vi "MotionMagicVoltage SetControl.vi"(0 "LimitReverseMotion":bool, 1 "FeedForward":dbl, 2 "OverrideBrakeDurNeutral":bool, 3 "Update Frequency (Hz)":dbl=100.0, 5 "StopSendingOtherRequests":bool=TRUE, 7 "Position":dbl, 9 "EnableFOC":bool=TRUE, 12 "Slot":i32, 13 "LimitForwardMotion":bool) -> (4 "DeviceReference Out":T1)   [LabVIEW 2023]
doc: "Requests Motion Magic® to target a final position using a motion profile. Users can optionally provide a voltage feedforward.\nMotion Magic® produces a motion profile in real-time while attempting to honor the Cruise Velocity, Acceleration, and Jerk value specified via the Motion Magic® configuration values. This control mode does not use the Expo_kV or Expo_kA configs. Target position can be changed on-the-fly and Motion Magic® will do its best to adjust the profile. This control mode is voltage-based, so relevant closed-loop gains will use Volts for the numerator."
uses:
  Users/Cory/Documents/PhoenixPro-LabVIEW-Generation/controls/DeviceReference.ctl
panel:
  in  "DeviceReference":T1
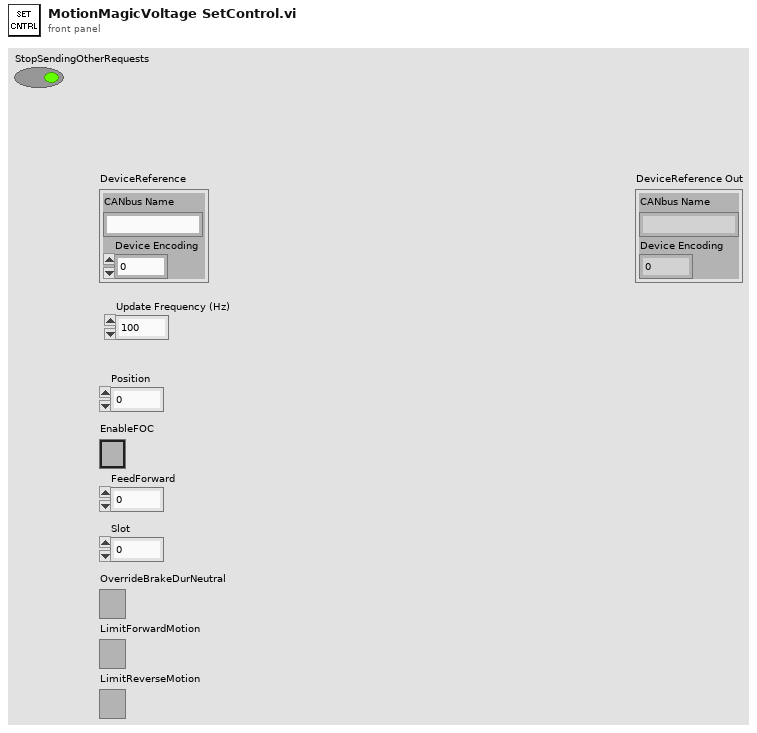
[diagram p1: front panel]
types:
  T1 = typedef "DeviceReference.ctl" = cluster{"CANbus Name":string, "Device Encoding":u32}
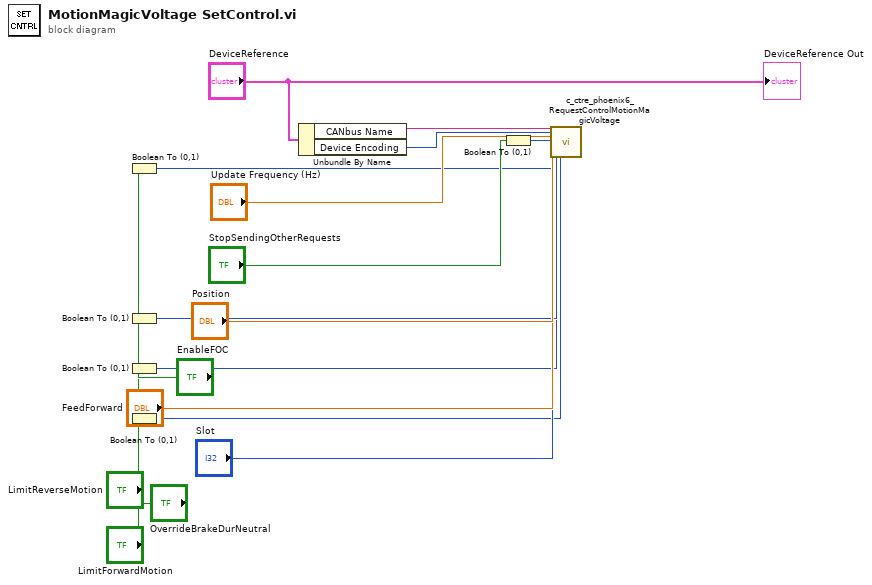
[diagram p0: block diagram]
diagram:
  n1 = Boolean To (0,1)(Boolean="EnableFOC") -> (0, 1=w9:i16)
  n2 = Boolean To (0,1)(Boolean="OverrideBrakeDurNeutral") -> (0, 1=w5:i16)
  n3 = Boolean To (0,1)(Boolean="LimitForwardMotion") -> (0, 1=w3:i16)
  n4 = Boolean To (0,1)(Boolean="LimitReverseMotion") -> (0, 1=w1:i16)
  n5 = Unbundle By Name("DeviceReference") -> ("CANbus Name"=w16:string, "Device Encoding"=w15:u32)
  n6 = Boolean To (0,1)(Boolean="StopSendingOtherRequests") -> (0, 1=w12:i16)
  n7 = call <vilib>:"c_ctre_phoenix6_RequestControlMotionMagicVoltage.vi"("String 2"=w16, "Numeric 2"=w15, "Numeric 3"="Update Frequency (Hz)", "Numeric 4"=w12, "Numeric 5"="Position", "Numeric 6"=w9, "Numeric 7"="FeedForward", "Numeric 8"="Slot", "Numeric 9"=w5, "Numeric 10"=w3, "Numeric 11"=w1) -> ()  [unwired: 15 in, 2 out]
  "DeviceReference Out" <- "DeviceReference"
